vi "_r2aio_32bit_8in_canopen_master.vi"() -> ()   [LabVIEW 2011]
panel:
  out "ret write_device_object_sdo INT":i16
  out "ret write_pdo_mapping 16":i16
  out "ret write_pdo_mapping 15":i16
  out "ret write_pdo_mapping 4":i16
  out "ret write_pdo_mapping 3":i16
  out "Analogue IN 8":i32
  out "ret read_node_object_dictionary 8":i16
  out "Analogue IN 7":i32
  out "ret read_node_object_dictionary 7":i16
  out "Analogue IN 6":i32
  out "ret read_node_object_dictionary 6":i16
  out "Analogue IN 5":i32
  out "ret read_node_object_dictionary 5":i16
  out "Analogue IN 4":i32
  out "ret read_node_object_dictionary 4":i16
  out "Analogue IN 3":i32
  out "ret read_node_object_dictionary 3":i16
  out "Analogue IN 2":i32
  out "ret read_node_object_dictionary 2":i16
  out "Analogue IN 1":i32
  out "ret write_pdo_mapping 14":i16
  out "ret write_pdo_mapping 13":i16
  out "ret write_pdo_mapping 12":i16
  out "ret write_pdo_mapping 11":i16
  out "ret write_pdo_mapping 10":i16
  out "ret write_pdo_mapping 9":i16
  out "ret write_pdo_mapping 8":i16
  out "ret write_pdo_mapping 7":i16
  out "ret write_pdo_mapping 6":i16
  out "ret write_pdo_mapping 2":i16
  out "ret add_node_object_dictionary 6402-8":i16
  out "ret add_node_object_dictionary 6402-7":i16
  out "ret add_node_object_dictionary 6402-6":i16
  out "ret add_node_object_dictionary 6402-5":i16
  out "ret add_node_object_dictionary 6402-4":i16
  out "ret add_node_object_dictionary 6402-3":i16
  out "ret add_node_object_dictionary 6402-2":i16
  out "datasize":u32
  out "Manufacturer software ver":string
  out "ret read_device_object_sdo 3":i16
  out "datasize":u32
  out "Manufacturer hardware ver":string
  out "ret read_device_object_sdo 2":i16
  out "datasize":u32
  out "Manufacturer dev name":string
  out "ret read_device_object_sdo 1":i16
  out "ret read_node_object_dictionary 1":i16
  in  "stop monitor":bool
  out "ret write_master_hbt":i16
  out "ret stop_can_master":i16
  out "ret write_pdo_mapping 5":i16
  out "ret write_pdo_mapping 1":i16
  out "ret add_node_object_dictionary 6402-1":i16
  out "ret write_device_object_sdo HBT":i16
  in  "slave node":u8
  in  "baudrate":T1(ring)
  in  "net":u8
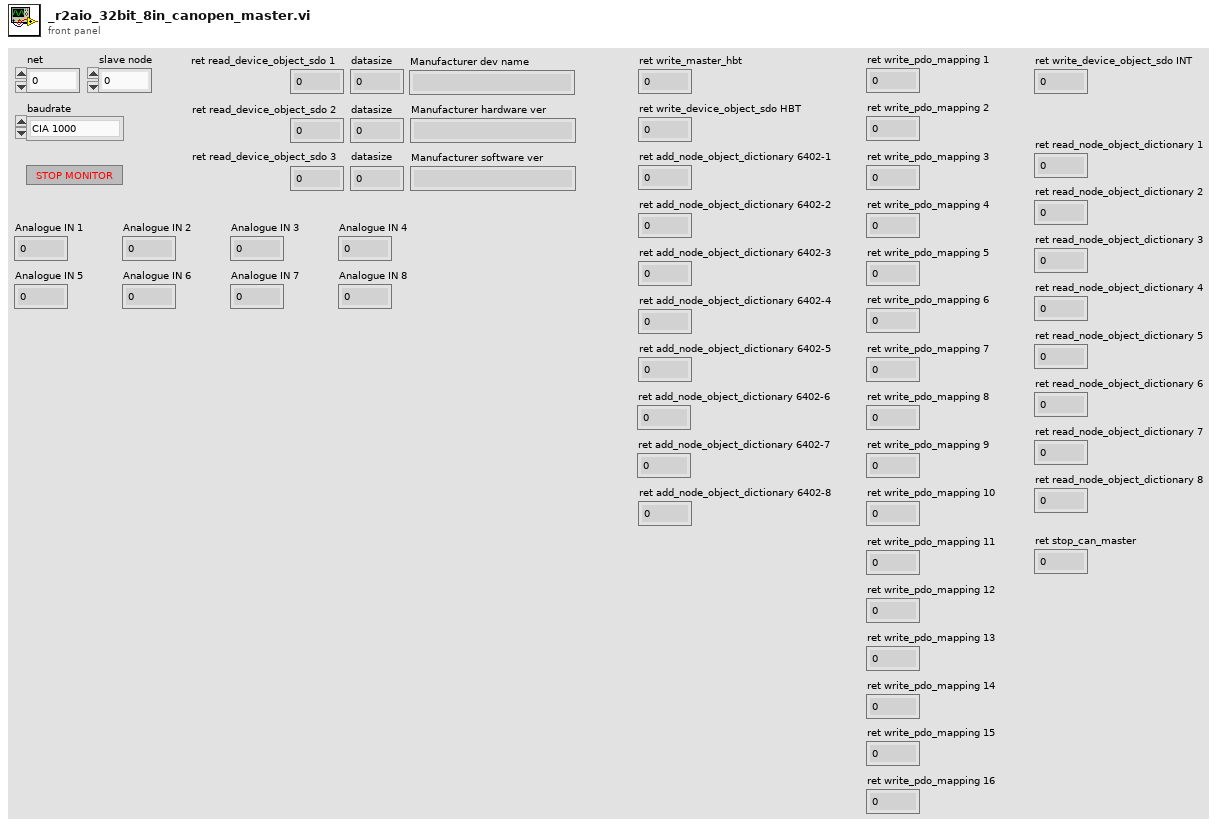
[diagram p1: front panel]
types:
  T1 = enum8{"CIA 1000", "CIA 800", "CIA 500", "CIA 250", "CIA 125", "CIA 100", "CIA 50", "CIA 20", "CIA 10", "CIA AUTO"}
diagram:
  n1 = flat-sequence {
    tunnel: ["slave node"] -> w51
    tunnel: w51 -> [w61]
    tunnel: [w61] -> w50
    tunnel: w50 -> [w63]
    tunnel: [w63] -> w53
    tunnel: w53 -> [w70]
    tunnel: [w70] -> w52
    tunnel: w52 -> [w73]
    tunnel: [w73] -> w46
    tunnel: w46 -> [w78]
    tunnel: [w78] -> w45
    tunnel: w45 -> [w83]
    tunnel: [w83] -> w44
    tunnel: w44 -> [w88]
    tunnel: [w88] -> w43
    tunnel: w43 -> [w93]
    tunnel: [w93] -> w42
    tunnel: w42 -> [w98]
    tunnel: [w98] -> w41
    tunnel: w41 -> [w103]
    tunnel: [w103] -> w40
    tunnel: w40 -> [w108]
    tunnel: [w108] -> w9
    tunnel: [w113] -> w49
    tunnel: w9 -> [w113]
    tunnel: [w118] -> w39
    tunnel: w49 -> [w118]
    tunnel: [w115] -> w24
    tunnel: w39 -> [w128]
    tunnel: [w128] -> w27
    tunnel: w24 -> [w126]
    tunnel: [w126] -> w23
    tunnel: w27 -> [w134]
    tunnel: [w134] -> w26
    tunnel: w23 -> [w133]
    tunnel: [w133] -> w22
    tunnel: w26 -> [w141]
    tunnel: [w141] -> w25
    tunnel: w22 -> [w140]
    tunnel: [w140] -> w21
    tunnel: [w149] -> w38
    tunnel: w25 -> [w149]
    tunnel: w21 -> [w147]
    tunnel: [w147] -> w20
    tunnel: w38 -> [w156]
    tunnel: [w156] -> w37
    tunnel: w20 -> [w154]
    tunnel: [w154] -> w19
    tunnel: w37 -> [w162]
    tunnel: [w162] -> w36
    tunnel: w19 -> [w161]
    tunnel: [w161] -> w18
    tunnel: w36 -> [w170]
    tunnel: [w170] -> w35
    tunnel: w18 -> [w168]
    tunnel: [w168] -> w17
    tunnel: w35 -> [w176]
    tunnel: [w176] -> w34
    tunnel: w17 -> [w175]
    tunnel: [w175] -> w16
    tunnel: w34 -> [w184]
    tunnel: [w184] -> w33
    tunnel: w16 -> [w182]
    tunnel: [w182] -> w15
    tunnel: w33 -> [w190]
    tunnel: [w190] -> w32
    tunnel: w15 -> [w189]
    tunnel: [w189] -> w14
    tunnel: w32 -> [w197]
    tunnel: [w197] -> w31
    tunnel: w14 -> [w196]
    tunnel: [w196] -> w13
    tunnel: w31 -> [w205]
    tunnel: [w205] -> w30
    tunnel: w13 -> [w203]
    tunnel: [w203] -> w12
    tunnel: w30 -> [w212]
    tunnel: [w212] -> w29
    tunnel: w12 -> [w210]
    tunnel: [w210] -> w11
    tunnel: w29 -> [w219]
    tunnel: [w219] -> w28
    tunnel: w11 -> [w217]
    tunnel: [w217] -> w10
    tunnel: [w225] -> w48
    tunnel: w28 -> [w225]
    tunnel: w10 -> [w224]
    tunnel: w48 -> [w237]
    tunnel: [w237] -> w47
    tunnel: [w239] -> w5
    tunnel: w47 -> [w239]
    tunnel: [w247] -> w7
    tunnel: w5 -> [w247]
    tunnel: w7 -> [w249]
    tunnel: [w249] -> w6
    tunnel: w6 -> [w250]
    tunnel: [w250] -> w4
    tunnel: w4 -> [w259]
    tunnel: [w259] -> w3
    tunnel: w3 -> [w260]
    tunnel: [w260] -> w2
    tunnel: w2 -> [w269]
    tunnel: [w269] -> w1
    tunnel: w1 -> [w271]
    tunnel: [w271] -> w8
    tunnel: w8 -> [w272]
    frame #0 {
      # "Start CAN master"
      n2 = call "start_can_master.vi"("br"="baudrate", "net"="net") -> ("return"=w57:i16)  [unwired: 9 in]
      n3 = Not Equal To 0?(x=w57) -> (x != 0?=w56:bool)
      n4 = Stop(stop? (T)=w56) -> ()
    }
    frame #1 {
      w59 = u8 129 items=["CAN_NMT_CS_DUMMY"=0, "CAN_NMT_START_REMOTE_NODE"=1, "CAN_NMT_STOP_REMOTE_NODE"=2, "CAN_NMT_ENTER_PRE_OPERATIONAL"=128, "CAN_NMT_RESET_NODE"=129, "CAN_NMT_RESET_COMMUNICATION"=130]  # NMT spec
      # "NMT Reset node"
      n5 = call "nmt_master_command.vi"("node"="slave node", "cs"=w59) -> ()  [unwired: 10 in]
    }
    frame #2 {
      n6 = Wait (ms)(milliseconds to wait=u32 500) -> ()  [unwired: 1 out]
    }
    frame #3 {
      # "Configure MASTER Heartbeat"
      n7 = call "write_master_hbt.vi"("hbt"=u16 1200, "node"=w63) -> ("return"=→"ret write_master_hbt":i16)  [unwired: 9 in]
    }
    frame #4 {
      # "Configure SLAVE Heartbeat"
      n8 = Build Array(u8 232, u8 3) -> (w66:u8[])
      n9 = call "write_device_object_sdo.vi"("node"=w70, "index"=u16 4119, "subind"=u8 0, "data"=w66, "datasize"=u32 2) -> ("return"=→"ret write_device_object_sdo HBT":i16)  [unwired: 10 in]
    }
    frame #5 {
      w75 = u16 4 items=["CAN_DEFTYPE_BOOLEAN"=1, "CAN_DEFTYPE_INTEGER8"=2, "CAN_DEFTYPE_INTEGER16"=3, "CAN_DEFTYPE_INTEGER32"=4, "CAN_DEFTYPE_UNSIGNED8"=5, "CAN_DEFTYPE_UNSIGNED16"=6, "CAN_DEFTYPE_UNSIGNED32"=7, "CAN_DEFTYPE_REAL32"=8, "CAN_DEFTYPE_VISIBLE_STRING"=9, "CAN_DEFTYPE_OCTET_STRING"=10, "CAN_DEFTYPE_UNICODE_STRING"=11, "CAN_DEFTYPE_TIME_OF_DAY"=12, "CAN_DEFTYPE_TIME_DIFFERENCE"=13, "CAN_DEFTYPE_DOMAIN"=15, "CAN_DEFTYPE_INTEGER24"=16, "CAN_DEFTYPE_REAL64"=17, "CAN_DEFTYPE_INTEGER40"=18, "CAN_DEFTYPE_INTEGER48"=19, "CAN_DEFTYPE_INTEGER56"=20, "CAN_DEFTYPE_INTEGER64"=21, "CAN_DEFTYPE_UNSIGNED24"=22, "CAN_DEFTYPE_UNSIGNED40"=24, "CAN_DEFTYPE_UNSIGNED48"=25, "CAN_DEFTYPE_UNSIGNED56"=26, "CAN_DEFTYPE_UNSIGNED64"=27]  # Data type spec
      # "Add Read Analogue input 1 object to MASTER dictionary"
      n10 = call "add_node_object_dictionary.vi"("type"=w75, "subind"=u8 1, "index"=u16 25602, "node"=w73) -> ("return"=→"ret add_node_object_dictionary 6402-1":i16)  [unwired: 7 in]
    }
    frame #6 {
      w80 = u16 4 items=["CAN_DEFTYPE_BOOLEAN"=1, "CAN_DEFTYPE_INTEGER8"=2, "CAN_DEFTYPE_INTEGER16"=3, "CAN_DEFTYPE_INTEGER32"=4, "CAN_DEFTYPE_UNSIGNED8"=5, "CAN_DEFTYPE_UNSIGNED16"=6, "CAN_DEFTYPE_UNSIGNED32"=7, "CAN_DEFTYPE_REAL32"=8, "CAN_DEFTYPE_VISIBLE_STRING"=9, "CAN_DEFTYPE_OCTET_STRING"=10, "CAN_DEFTYPE_UNICODE_STRING"=11, "CAN_DEFTYPE_TIME_OF_DAY"=12, "CAN_DEFTYPE_TIME_DIFFERENCE"=13, "CAN_DEFTYPE_DOMAIN"=15, "CAN_DEFTYPE_INTEGER24"=16, "CAN_DEFTYPE_REAL64"=17, "CAN_DEFTYPE_INTEGER40"=18, "CAN_DEFTYPE_INTEGER48"=19, "CAN_DEFTYPE_INTEGER56"=20, "CAN_DEFTYPE_INTEGER64"=21, "CAN_DEFTYPE_UNSIGNED24"=22, "CAN_DEFTYPE_UNSIGNED40"=24, "CAN_DEFTYPE_UNSIGNED48"=25, "CAN_DEFTYPE_UNSIGNED56"=26, "CAN_DEFTYPE_UNSIGNED64"=27]  # Data type spec
      # "Add Read Analogue input 2 object to MASTER dictionary"
      n11 = call "add_node_object_dictionary.vi"("type"=w80, "subind"=u8 2, "index"=u16 25602, "node"=w78) -> ("return"=→"ret add_node_object_dictionary 6402-2":i16)  [unwired: 7 in]
    }
    frame #7 {
      w85 = u16 4 items=["CAN_DEFTYPE_BOOLEAN"=1, "CAN_DEFTYPE_INTEGER8"=2, "CAN_DEFTYPE_INTEGER16"=3, "CAN_DEFTYPE_INTEGER32"=4, "CAN_DEFTYPE_UNSIGNED8"=5, "CAN_DEFTYPE_UNSIGNED16"=6, "CAN_DEFTYPE_UNSIGNED32"=7, "CAN_DEFTYPE_REAL32"=8, "CAN_DEFTYPE_VISIBLE_STRING"=9, "CAN_DEFTYPE_OCTET_STRING"=10, "CAN_DEFTYPE_UNICODE_STRING"=11, "CAN_DEFTYPE_TIME_OF_DAY"=12, "CAN_DEFTYPE_TIME_DIFFERENCE"=13, "CAN_DEFTYPE_DOMAIN"=15, "CAN_DEFTYPE_INTEGER24"=16, "CAN_DEFTYPE_REAL64"=17, "CAN_DEFTYPE_INTEGER40"=18, "CAN_DEFTYPE_INTEGER48"=19, "CAN_DEFTYPE_INTEGER56"=20, "CAN_DEFTYPE_INTEGER64"=21, "CAN_DEFTYPE_UNSIGNED24"=22, "CAN_DEFTYPE_UNSIGNED40"=24, "CAN_DEFTYPE_UNSIGNED48"=25, "CAN_DEFTYPE_UNSIGNED56"=26, "CAN_DEFTYPE_UNSIGNED64"=27]  # Data type spec
      # "Add Read Analogue input 3 object to MASTER dictionary"
      n12 = call "add_node_object_dictionary.vi"("type"=w85, "subind"=u8 3, "index"=u16 25602, "node"=w83) -> ("return"=→"ret add_node_object_dictionary 6402-3":i16)  [unwired: 7 in]
    }
    frame #8 {
      w90 = u16 4 items=["CAN_DEFTYPE_BOOLEAN"=1, "CAN_DEFTYPE_INTEGER8"=2, "CAN_DEFTYPE_INTEGER16"=3, "CAN_DEFTYPE_INTEGER32"=4, "CAN_DEFTYPE_UNSIGNED8"=5, "CAN_DEFTYPE_UNSIGNED16"=6, "CAN_DEFTYPE_UNSIGNED32"=7, "CAN_DEFTYPE_REAL32"=8, "CAN_DEFTYPE_VISIBLE_STRING"=9, "CAN_DEFTYPE_OCTET_STRING"=10, "CAN_DEFTYPE_UNICODE_STRING"=11, "CAN_DEFTYPE_TIME_OF_DAY"=12, "CAN_DEFTYPE_TIME_DIFFERENCE"=13, "CAN_DEFTYPE_DOMAIN"=15, "CAN_DEFTYPE_INTEGER24"=16, "CAN_DEFTYPE_REAL64"=17, "CAN_DEFTYPE_INTEGER40"=18, "CAN_DEFTYPE_INTEGER48"=19, "CAN_DEFTYPE_INTEGER56"=20, "CAN_DEFTYPE_INTEGER64"=21, "CAN_DEFTYPE_UNSIGNED24"=22, "CAN_DEFTYPE_UNSIGNED40"=24, "CAN_DEFTYPE_UNSIGNED48"=25, "CAN_DEFTYPE_UNSIGNED56"=26, "CAN_DEFTYPE_UNSIGNED64"=27]  # Data type spec
      # "Add Read Analogue input 4 object to MASTER dictionary"
      n13 = call "add_node_object_dictionary.vi"("type"=w90, "subind"=u8 4, "index"=u16 25602, "node"=w88) -> ("return"=→"ret add_node_object_dictionary 6402-4":i16)  [unwired: 7 in]
    }
    frame #9 {
      w95 = u16 4 items=["CAN_DEFTYPE_BOOLEAN"=1, "CAN_DEFTYPE_INTEGER8"=2, "CAN_DEFTYPE_INTEGER16"=3, "CAN_DEFTYPE_INTEGER32"=4, "CAN_DEFTYPE_UNSIGNED8"=5, "CAN_DEFTYPE_UNSIGNED16"=6, "CAN_DEFTYPE_UNSIGNED32"=7, "CAN_DEFTYPE_REAL32"=8, "CAN_DEFTYPE_VISIBLE_STRING"=9, "CAN_DEFTYPE_OCTET_STRING"=10, "CAN_DEFTYPE_UNICODE_STRING"=11, "CAN_DEFTYPE_TIME_OF_DAY"=12, "CAN_DEFTYPE_TIME_DIFFERENCE"=13, "CAN_DEFTYPE_DOMAIN"=15, "CAN_DEFTYPE_INTEGER24"=16, "CAN_DEFTYPE_REAL64"=17, "CAN_DEFTYPE_INTEGER40"=18, "CAN_DEFTYPE_INTEGER48"=19, "CAN_DEFTYPE_INTEGER56"=20, "CAN_DEFTYPE_INTEGER64"=21, "CAN_DEFTYPE_UNSIGNED24"=22, "CAN_DEFTYPE_UNSIGNED40"=24, "CAN_DEFTYPE_UNSIGNED48"=25, "CAN_DEFTYPE_UNSIGNED56"=26, "CAN_DEFTYPE_UNSIGNED64"=27]  # Data type spec
      # "Add Read Analogue input 5 object to MASTER dictionary"
      n14 = call "add_node_object_dictionary.vi"("type"=w95, "subind"=u8 5, "index"=u16 25602, "node"=w93) -> ("return"=→"ret add_node_object_dictionary 6402-5":i16)  [unwired: 7 in]
    }
    frame #10 {
      w100 = u16 4 items=["CAN_DEFTYPE_BOOLEAN"=1, "CAN_DEFTYPE_INTEGER8"=2, "CAN_DEFTYPE_INTEGER16"=3, "CAN_DEFTYPE_INTEGER32"=4, "CAN_DEFTYPE_UNSIGNED8"=5, "CAN_DEFTYPE_UNSIGNED16"=6, "CAN_DEFTYPE_UNSIGNED32"=7, "CAN_DEFTYPE_REAL32"=8, "CAN_DEFTYPE_VISIBLE_STRING"=9, "CAN_DEFTYPE_OCTET_STRING"=10, "CAN_DEFTYPE_UNICODE_STRING"=11, "CAN_DEFTYPE_TIME_OF_DAY"=12, "CAN_DEFTYPE_TIME_DIFFERENCE"=13, "CAN_DEFTYPE_DOMAIN"=15, "CAN_DEFTYPE_INTEGER24"=16, "CAN_DEFTYPE_REAL64"=17, "CAN_DEFTYPE_INTEGER40"=18, "CAN_DEFTYPE_INTEGER48"=19, "CAN_DEFTYPE_INTEGER56"=20, "CAN_DEFTYPE_INTEGER64"=21, "CAN_DEFTYPE_UNSIGNED24"=22, "CAN_DEFTYPE_UNSIGNED40"=24, "CAN_DEFTYPE_UNSIGNED48"=25, "CAN_DEFTYPE_UNSIGNED56"=26, "CAN_DEFTYPE_UNSIGNED64"=27]  # Data type spec
      # "Add Read Analogue input 6 object to MASTER dictionary"
      n15 = call "add_node_object_dictionary.vi"("type"=w100, "subind"=u8 6, "index"=u16 25602, "node"=w98) -> ("return"=→"ret add_node_object_dictionary 6402-6":i16)  [unwired: 7 in]
    }
    frame #11 {
      w105 = u16 4 items=["CAN_DEFTYPE_BOOLEAN"=1, "CAN_DEFTYPE_INTEGER8"=2, "CAN_DEFTYPE_INTEGER16"=3, "CAN_DEFTYPE_INTEGER32"=4, "CAN_DEFTYPE_UNSIGNED8"=5, "CAN_DEFTYPE_UNSIGNED16"=6, "CAN_DEFTYPE_UNSIGNED32"=7, "CAN_DEFTYPE_REAL32"=8, "CAN_DEFTYPE_VISIBLE_STRING"=9, "CAN_DEFTYPE_OCTET_STRING"=10, "CAN_DEFTYPE_UNICODE_STRING"=11, "CAN_DEFTYPE_TIME_OF_DAY"=12, "CAN_DEFTYPE_TIME_DIFFERENCE"=13, "CAN_DEFTYPE_DOMAIN"=15, "CAN_DEFTYPE_INTEGER24"=16, "CAN_DEFTYPE_REAL64"=17, "CAN_DEFTYPE_INTEGER40"=18, "CAN_DEFTYPE_INTEGER48"=19, "CAN_DEFTYPE_INTEGER56"=20, "CAN_DEFTYPE_INTEGER64"=21, "CAN_DEFTYPE_UNSIGNED24"=22, "CAN_DEFTYPE_UNSIGNED40"=24, "CAN_DEFTYPE_UNSIGNED48"=25, "CAN_DEFTYPE_UNSIGNED56"=26, "CAN_DEFTYPE_UNSIGNED64"=27]  # Data type spec
      # "Add Read Analogue input 7 object to MASTER dictionary"
      n16 = call "add_node_object_dictionary.vi"("type"=w105, "subind"=u8 7, "index"=u16 25602, "node"=w103) -> ("return"=→"ret add_node_object_dictionary 6402-7":i16)  [unwired: 7 in]
    }
    frame #12 {
      w110 = u16 4 items=["CAN_DEFTYPE_BOOLEAN"=1, "CAN_DEFTYPE_INTEGER8"=2, "CAN_DEFTYPE_INTEGER16"=3, "CAN_DEFTYPE_INTEGER32"=4, "CAN_DEFTYPE_UNSIGNED8"=5, "CAN_DEFTYPE_UNSIGNED16"=6, "CAN_DEFTYPE_UNSIGNED32"=7, "CAN_DEFTYPE_REAL32"=8, "CAN_DEFTYPE_VISIBLE_STRING"=9, "CAN_DEFTYPE_OCTET_STRING"=10, "CAN_DEFTYPE_UNICODE_STRING"=11, "CAN_DEFTYPE_TIME_OF_DAY"=12, "CAN_DEFTYPE_TIME_DIFFERENCE"=13, "CAN_DEFTYPE_DOMAIN"=15, "CAN_DEFTYPE_INTEGER24"=16, "CAN_DEFTYPE_REAL64"=17, "CAN_DEFTYPE_INTEGER40"=18, "CAN_DEFTYPE_INTEGER48"=19, "CAN_DEFTYPE_INTEGER56"=20, "CAN_DEFTYPE_INTEGER64"=21, "CAN_DEFTYPE_UNSIGNED24"=22, "CAN_DEFTYPE_UNSIGNED40"=24, "CAN_DEFTYPE_UNSIGNED48"=25, "CAN_DEFTYPE_UNSIGNED56"=26, "CAN_DEFTYPE_UNSIGNED64"=27]  # Data type spec
      # "Add Read Analogue input 8 object to MASTER dictionary"
      n17 = call "add_node_object_dictionary.vi"("type"=w110, "subind"=u8 8, "index"=u16 25602, "node"=w108) -> ("return"=→"ret add_node_object_dictionary 6402-8":i16)  [unwired: 7 in]
    }
    frame #13 {
      w114 = u8 1 items=["CAN_NMT_CS_DUMMY"=0, "CAN_NMT_START_REMOTE_NODE"=1, "CAN_NMT_STOP_REMOTE_NODE"=2, "CAN_NMT_ENTER_PRE_OPERATIONAL"=128, "CAN_NMT_RESET_NODE"=129, "CAN_NMT_RESET_COMMUNICATION"=130]  # NMT spec
      # "NMT Start remote node"
      n18 = call "nmt_master_command.vi"("node"=w113, "cs"=w114) -> ()  [unwired: 10 in]
    }
    frame #14 {
      # "Disable RPDO1 mapping"
      n19 = Subtract(x=w118, y=u8 1) -> (x-y=w117:u8)
      n20 = Multiply(x=w117, y=u8 4) -> (x*y=w116:u8)
      n21 = To Unsigned Word Integer(number=w116) -> (unsigned 16bit integer=w115:u16)
      n22 = Add(x=w115, y=u16 5632) -> (x+y=w121:u16)
      n23 = call "write_pdo_mapping.vi"("data"=u32 0, "subind"=u8 0, "index"=w121) -> ("return"=→"ret write_pdo_mapping 1":i16)  [unwired: 8 in]
    }
    frame #15 {
      # "Disable RPDO2 mapping"
      n24 = Add(x=w126, y=u16 5633) -> (x+y=w127:u16)
      n25 = call "write_pdo_mapping.vi"("data"=u32 0, "subind"=u8 0, "index"=w127) -> ("return"=→"ret write_pdo_mapping 2":i16)  [unwired: 8 in]
    }
    frame #16 {
      # "Disable RPDO3 mapping"
      n26 = Add(x=w133, y=u16 5634) -> (x+y=w135:u16)
      n27 = call "write_pdo_mapping.vi"("data"=u32 0, "subind"=u8 0, "index"=w135) -> ("return"=→"ret write_pdo_mapping 3":i16)  [unwired: 8 in]
    }
    frame #17 {
      # "Disable RPDO4 mapping"
      n28 = Add(x=w140, y=u16 5635) -> (x+y=w142:u16)
      n29 = call "write_pdo_mapping.vi"("data"=u32 0, "subind"=u8 0, "index"=w142) -> ("return"=→"ret write_pdo_mapping 4":i16)  [unwired: 8 in]
    }
    frame #18 {
      # "Map Read Analogue Input 1 RPDO1"
      n30 = Add(x=w147, y=u16 5632) -> (x+y=w148:u16)
      n31 = call "write_pdo_mapping.vi"("data"=u32 1677852960, "subind"=u8 1, "index"=w148) -> ("return"=→"ret write_pdo_mapping 5":i16)  [unwired: 8 in]
    }
    frame #19 {
      # "Map Read Analogue Input 2 RPDO1"
      n32 = Add(x=w154, y=u16 5632) -> (x+y=w155:u16)
      n33 = call "write_pdo_mapping.vi"("data"=u32 1677853216, "subind"=u8 2, "index"=w155) -> ("return"=→"ret write_pdo_mapping 6":i16)  [unwired: 8 in]
    }
    frame #20 {
      # "Map Read Analogue Input 3 RPDO2"
      n34 = Add(x=w161, y=u16 5633) -> (x+y=w164:u16)
      n35 = call "write_pdo_mapping.vi"("data"=u32 1677853472, "subind"=u8 1, "index"=w164) -> ("return"=→"ret write_pdo_mapping 7":i16)  [unwired: 8 in]
    }
    frame #21 {
      # "Map Read Analogue Input 4 RPDO2"
      n36 = Add(x=w168, y=u16 5633) -> (x+y=w169:u16)
      n37 = call "write_pdo_mapping.vi"("data"=u32 1677853728, "subind"=u8 2, "index"=w169) -> ("return"=→"ret write_pdo_mapping 8":i16)  [unwired: 8 in]
    }
    frame #22 {
      # "Map Read Analogue Input 5 RPDO3"
      n38 = Add(x=w175, y=u16 5634) -> (x+y=w177:u16)
      n39 = call "write_pdo_mapping.vi"("data"=u32 1677853984, "subind"=u8 1, "index"=w177) -> ("return"=→"ret write_pdo_mapping 9":i16)  [unwired: 8 in]
    }
    frame #23 {
      # "Map Read Analogue Input 6 RPDO3"
      n40 = Add(x=w182, y=u16 5634) -> (x+y=w183:u16)
      n41 = call "write_pdo_mapping.vi"("data"=u32 1677854240, "subind"=u8 2, "index"=w183) -> ("return"=→"ret write_pdo_mapping 10":i16)  [unwired: 8 in]
    }
    frame #24 {
      # "Map Read Analogue Input 7 RPDO4"
      n42 = Add(x=w189, y=u16 5635) -> (x+y=w192:u16)
      n43 = call "write_pdo_mapping.vi"("data"=u32 1677854496, "subind"=u8 1, "index"=w192) -> ("return"=→"ret write_pdo_mapping 11":i16)  [unwired: 8 in]
    }
    frame #25 {
      # "Map Read Analogue Input 8 RPDO4"
      n44 = Add(x=w196, y=u16 5635) -> (x+y=w199:u16)
      n45 = call "write_pdo_mapping.vi"("data"=u32 1677854752, "subind"=u8 2, "index"=w199) -> ("return"=→"ret write_pdo_mapping 12":i16)  [unwired: 8 in]
    }
    frame #26 {
      # "Enable RPDO1 mapping"
      n46 = Add(x=w203, y=u16 5632) -> (x+y=w204:u16)
      n47 = call "write_pdo_mapping.vi"("data"=u32 2, "subind"=u8 0, "index"=w204) -> ("return"=→"ret write_pdo_mapping 13":i16)  [unwired: 8 in]
    }
    frame #27 {
      # "Enable RPDO2 mapping"
      n48 = Add(x=w210, y=u16 5633) -> (x+y=w211:u16)
      n49 = call "write_pdo_mapping.vi"("data"=u32 2, "subind"=u8 0, "index"=w211) -> ("return"=→"ret write_pdo_mapping 14":i16)  [unwired: 8 in]
    }
    frame #28 {
      # "Enable RPDO3 mapping"
      n50 = Add(x=w217, y=u16 5634) -> (x+y=w218:u16)
      n51 = call "write_pdo_mapping.vi"("data"=u32 2, "subind"=u8 0, "index"=w218) -> ("return"=→"ret write_pdo_mapping 15":i16)  [unwired: 8 in]
    }
    frame #29 {
      # "Enable RPDO4 mapping"
      n52 = Add(x=w224, y=u16 5635) -> (x+y=w227:u16)
      n53 = call "write_pdo_mapping.vi"("data"=u32 2, "subind"=u8 0, "index"=w227) -> ("return"=→"ret write_pdo_mapping 16":i16)  [unwired: 8 in]
    }
    frame #30 {
      # "Enable GLOBAL interrupts"
      n54 = Build Array(u8 1) -> (w233:u8[])
      n55 = call "write_device_object_sdo.vi"("node"=w237, "index"=u16 25635, "subind"=u8 0, "data"=w233, "datasize"=u32 1) -> ("return"=→"ret write_device_object_sdo INT":i16)  [unwired: 10 in]
    }
    frame #31 {
      n56 = Wait (ms)(milliseconds to wait=u32 500) -> ()  [unwired: 1 out]
    }
    frame #32 {
      # "Read Manufacturer Device Name"
      n57 = call "read_device_object_sdo.vi"("node"=w247, "index"=u16 4104, "subind"=u8 0, "datasize"=u32 128) -> ("return"=→"ret read_device_object_sdo 1":i16, "data"=w242:u8[], "datasize"=→"datasize":u32)  [unwired: 9 in]
      n58 = Byte Array To String(unsigned byte array=w242) -> (string=→"Manufacturer dev name":string)
    }
    frame #33 {
      n59 = Wait (ms)(milliseconds to wait=u32 500) -> ()  [unwired: 1 out]
    }
    frame #34 {
      # "Read Manufacturer Hardware Version"
      n60 = call "read_device_object_sdo.vi"("node"=w250, "index"=u16 4105, "subind"=u8 0, "datasize"=u32 128) -> ("return"=→"ret read_device_object_sdo 2":i16, "data"=w253:u8[], "datasize"=→"datasize":u32)  [unwired: 9 in]
      n61 = Byte Array To String(unsigned byte array=w253) -> (string=→"Manufacturer hardware ver":string)
    }
    frame #35 {
      n62 = Wait (ms)(milliseconds to wait=u32 500) -> ()  [unwired: 1 out]
    }
    frame #36 {
      # "Read Manufacturer Software Version"
      n63 = call "read_device_object_sdo.vi"("node"=w260, "index"=u16 4106, "subind"=u8 0, "datasize"=u32 128) -> ("return"=→"ret read_device_object_sdo 3":i16, "data"=w263:u8[], "datasize"=→"datasize":u32)  [unwired: 9 in]
      n64 = Byte Array To String(unsigned byte array=w263) -> (string=→"Manufacturer software ver":string)
    }
    frame #37 {
      n65 = Wait (ms)(milliseconds to wait=u32 500) -> ()  [unwired: 1 out]
    }
    frame #38 {
      w270 = u8 1 items=["NOT_VALID", "VALID"]  # State
      # "Set all PDOs valid"
      n66 = call "set_all_pdos_state.vi"("state"=w270) -> ()  [unwired: 11 in]
    }
    frame #39 {
      # "Monitor"
      n67 = while {
        tunnel: w272 -> [w273]
        stop <- "stop monitor" stop-if-true
        n68 = call "read_node_object_dictionary.vi"("node"=w273, "index"=u16 25602, "subind"=u8 1) -> ("return"=→"ret read_node_object_dictionary 1":i16, "num"=w310:u64)  [unwired: 10 in, 1 out]
        n69 = To Long Integer(number=w310) -> (32bit integer=→"Analogue IN 1":i32)
        n70 = call "read_node_object_dictionary.vi"("node"=w273, "index"=u16 25602, "subind"=u8 2) -> ("return"=→"ret read_node_object_dictionary 2":i16, "num"=w305:u64)  [unwired: 10 in, 1 out]
        n71 = To Long Integer(number=w305) -> (32bit integer=→"Analogue IN 2":i32)
        n72 = call "read_node_object_dictionary.vi"("node"=w273, "index"=u16 25602, "subind"=u8 3) -> ("return"=→"ret read_node_object_dictionary 3":i16, "num"=w300:u64)  [unwired: 10 in, 1 out]
        n73 = To Long Integer(number=w300) -> (32bit integer=→"Analogue IN 3":i32)
        n74 = call "read_node_object_dictionary.vi"("node"=w273, "index"=u16 25602, "subind"=u8 4) -> ("return"=→"ret read_node_object_dictionary 4":i16, "num"=w295:u64)  [unwired: 10 in, 1 out]
        n75 = To Long Integer(number=w295) -> (32bit integer=→"Analogue IN 4":i32)
        n76 = call "read_node_object_dictionary.vi"("node"=w273, "index"=u16 25602, "subind"=u8 5) -> ("return"=→"ret read_node_object_dictionary 5":i16, "num"=w290:u64)  [unwired: 10 in, 1 out]
        n77 = To Long Integer(number=w290) -> (32bit integer=→"Analogue IN 5":i32)
        n78 = call "read_node_object_dictionary.vi"("node"=w273, "index"=u16 25602, "subind"=u8 6) -> ("return"=→"ret read_node_object_dictionary 6":i16, "num"=w285:u64)  [unwired: 10 in, 1 out]
        n79 = To Long Integer(number=w285) -> (32bit integer=→"Analogue IN 6":i32)
        n80 = call "read_node_object_dictionary.vi"("node"=w273, "index"=u16 25602, "subind"=u8 7) -> ("return"=→"ret read_node_object_dictionary 7":i16, "num"=w280:u64)  [unwired: 10 in, 1 out]
        n81 = To Long Integer(number=w280) -> (32bit integer=→"Analogue IN 7":i32)
        n82 = call "read_node_object_dictionary.vi"("node"=w273, "index"=u16 25602, "subind"=u8 8) -> ("return"=→"ret read_node_object_dictionary 8":i16, "num"=w275:u64)  [unwired: 10 in, 1 out]
        n83 = To Long Integer(number=w275) -> (32bit integer=→"Analogue IN 8":i32)
      }
    }
    frame #40 {
      # "Stop CAN master"
      n84 = call "stop_can_master.vi"() -> ("return"=→"ret stop_can_master":i16)  [unwired: 11 in]
    }
  }
